vi "GetUTDevOpenSts.vi"(8 "错误输入（无错误）":errorcluster, 11 "板卡序号":u8) -> (0 "错误输出":errorcluster, 3 "返回值":i32)   [LabVIEW 2014]
uses:
  ZXUTConfigMgr.dll
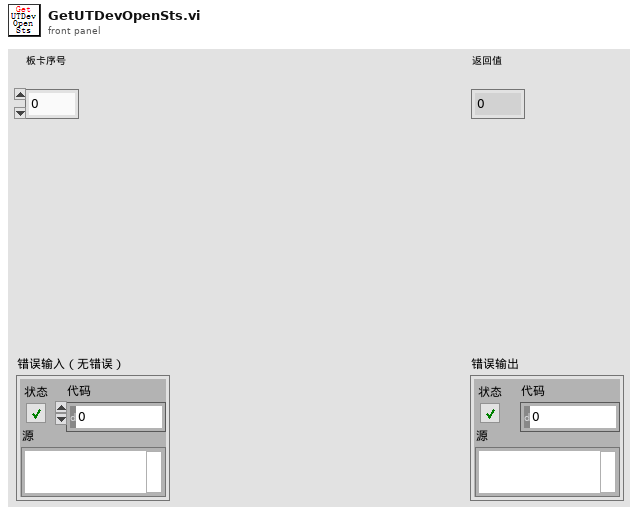
[diagram p1: front panel]
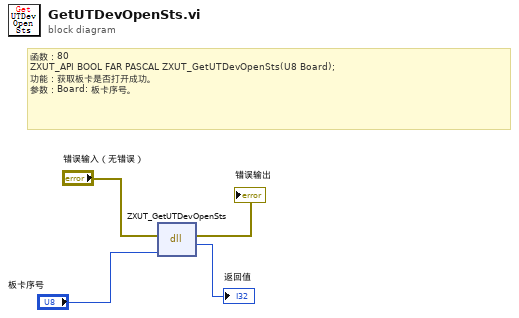
[diagram p0: block diagram]
diagram:
  # "函数：80\nZXUT_API BOOL\tFAR PASCAL ZXUT_GetUTDevOpenSts(U8 Board);\n功能：获取板卡是否打开成功。\n参数：Board: 板卡序号。"
  n1 = dll-call lib="PTH2eabs D软件超声实时监测软件ZXUTAppDemo(华南理工V02.00)X86DllZXUTConfigMgr.dll" fn="ZXUT_GetUTDevOpenSts"(error in="错误输入（无错误）", "Board"="板卡序号") -> (error out=→"错误输出":errorcluster, "返回值"=→"返回值":i32)  [unwired: 3 in, 1 out]
